vi "Get Unitless Values.vi"(8 "error in (no error)":errorcluster, 11 "Analyze Results Fluence in":refnum<class "Analyze Results Fluence.lvclass">) -> (0 "error out":errorcluster, 2 "UnitLess Values":T1[](array[typedef]), 3 "Analyze Results Fluence out":refnum<class "Analyze Results Fluence.lvclass">)   [LabVIEW 2020, in "Analyze Results Fluence.lvclass"]
uses:
  Analyze Results Fluence.lvclass
  Results Base/UnitLessValue.ctl
  Analyze Results Fluence.lvclass/Analyze Results Fluence.ctl
  Results Base/Analyze Results Base.lvclass
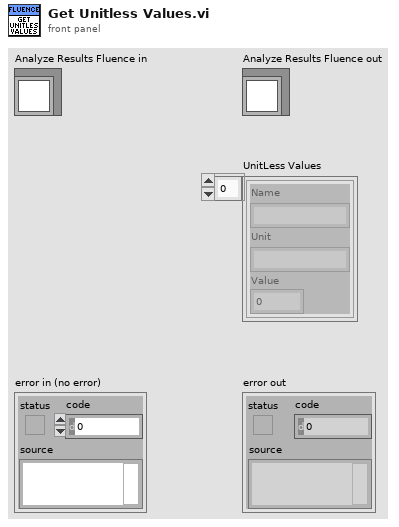
[diagram p1: front panel]
types:
  T1 = typedef "Analyze Results Base.lvclass/UnitLessValue.ctl" = cluster{"Name":string, "Unit":string, "Value":dbl}
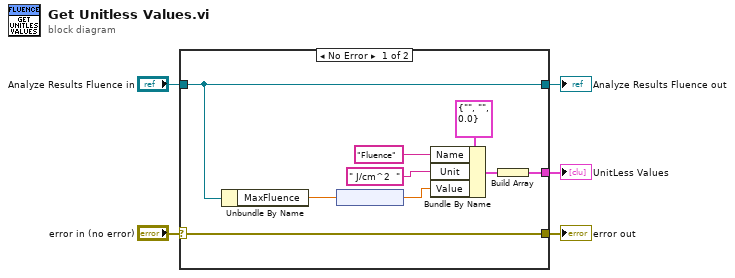
[diagram p0: block diagram]
diagram:
  n1 = case shown="No Error" "error in (no error)" {
    selector: "error in (no error)" -> [w11 w15]
    tunnel: "Analyze Results Fluence in" -> [w12 w16]
    tunnel: [w8 _] -> w2
    tunnel: [w12 w16] -> w3
    tunnel: [w11 w15] -> w1
    frame No Error {
      n2 = Unbundle By Name(w12) -> ("MaxFluence"=w6:dbl[unit])
      n3 = node(w6) -> (w7:dbl)
      n4 = Bundle By Name(cluster=T1 {"Name"="", "Unit"="", "Value"=0.0} ("UnitLessValue"), "Name"="Fluence", "Unit"=" J/cm^2  ", "Value"=w7) -> (w13:T1)
      n5 = Build Array(w13) -> (w8:T1[])
    }
    frame Error {
    }
  }
  "error out" <- w1
  "Analyze Results Fluence out" <- w3
  "UnitLess Values" <- w2
